vi "RegulatorMessageLoop.vi"(8 "Error In":errorcluster, 11 "CommunicationRefs":T1) -> (0 "Error Out":errorcluster)   [LabVIEW 2015]
uses:
  TypeDefs/CommunicationRefs.ctl
  TypeDefs/MessageCluster.ctl
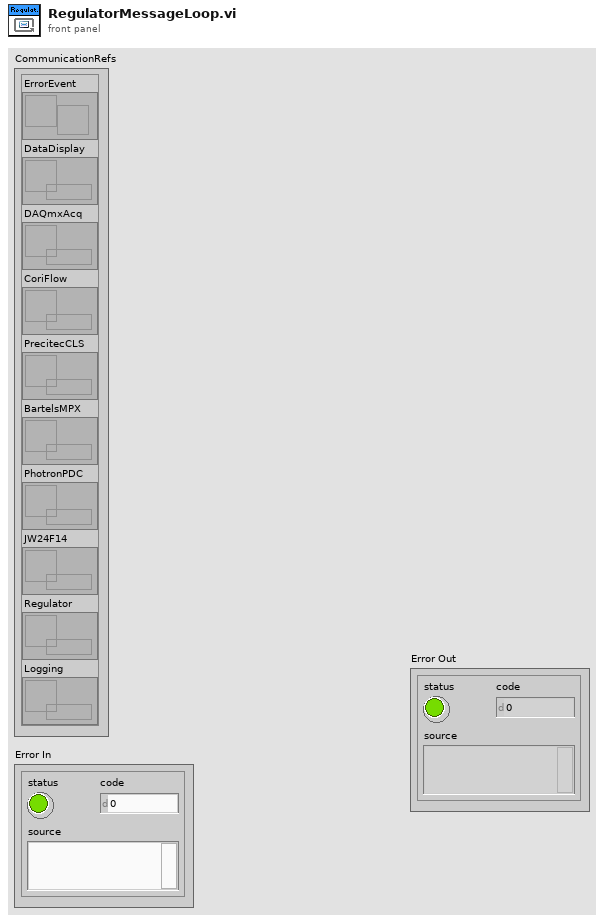
[diagram p1: front panel]
types:
  T1 = typedef "CommunicationRefs.ctl" = cluster{"ErrorEvent":refnum<user-event>, "DataDisplay":refnum<queue>, "DAQmxAcq":refnum<queue>, "CoriFlow":refnum<queue>, "PrecitecCLS":refnum<queue>, "BartelsMPX":refnum<queue>, "PhotronPDC":refnum<queue>, "JW24F14":refnum<queue>, "Regulator":refnum<queue>, "Logging":refnum<queue>}
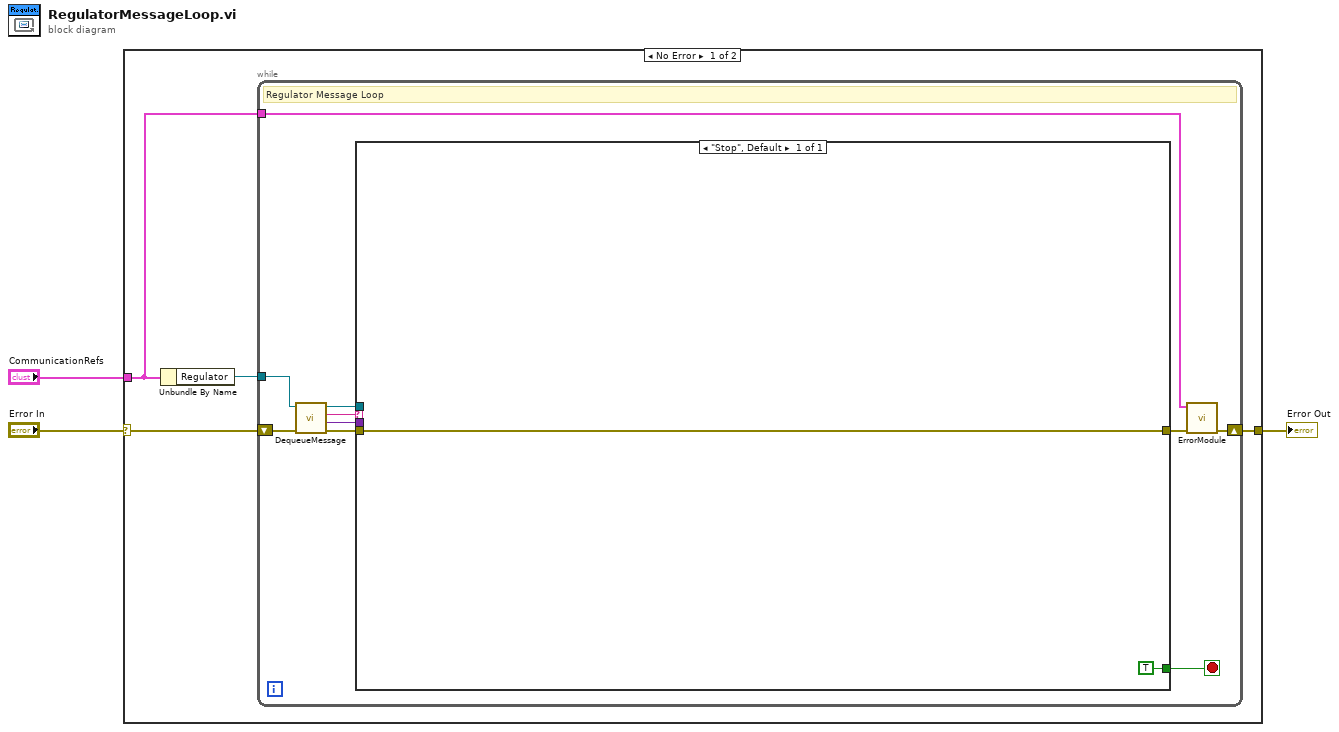
[diagram p0: block diagram]
diagram:
  n1 = case shown="No Error" "Error In" {
    selector: "Error In" -> [w7 w20]
    tunnel: [w6 w20] -> w2
    tunnel: "CommunicationRefs" -> [w5 _]
    frame No Error {
      n2 = Unbundle By Name(w5) -> ("Regulator"=w4:refnum<queue>)
      n3 = while {
        tunnel: w5 -> [w12]
        shift-right: [w13] -> w6
        shift-left: w7 -> [w17]
        tunnel: w4 -> [w9]
        stop <- w11 stop-if-true
        # "Regulator Message Loop"
        n4 = call "DequeueMessage.vi"("error in (no error)"=w17, "MessageQueue"=w9) -> ("error out"=w14:errorcluster, "MessageData"=w15:variant, "Message"=w16:string, "dupMessageQueue"=w8:refnum<queue>)  [unwired: 6 in]
        n5 = case shown="\"Stop\", Default" w16 {
          tunnel: w15 -> [_]
          tunnel: w14 -> [w18]
          tunnel: [TRUE] -> w11
          tunnel: [w18] -> w10
          tunnel: w8 -> [_]
          frame "Stop", Default {
          }
        }
        n6 = call "ErrorModule.vi"("Error In"=w10, "CommunicationRefs"=w12) -> ("Error Out"=w13:errorcluster)  [unwired: 9 in]
      }
    }
    frame Error {
    }
  }
  "Error Out" <- w2
